vi "Pick Up Order.vi"(8 "error in (no error)":errorcluster, 10 "Beverage":refnum<class "Beverage.lvclass">, 11 "Stub Pick Up Order In":refnum<class "Stub Pick Up Order.lvclass">) -> (0 "error out":errorcluster, 3 "Stub Pick Up Order Out":refnum<class "Stub Pick Up Order.lvclass">)   [LabVIEW 2020, in "Stub Pick Up Order.lvclass"]
uses:
  Stub Pick Up Order.lvclass
  Support/Beverages/Beverage/Beverage.lvclass
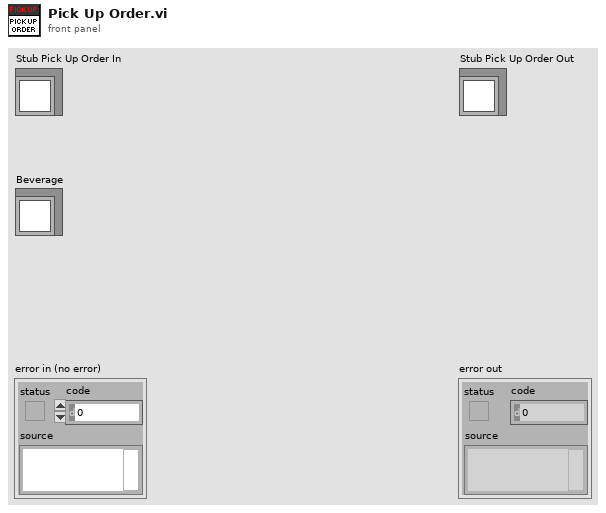
[diagram p1: front panel]
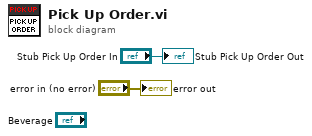
[diagram p0: block diagram]
diagram:
  "error out" <- "error in (no error)"
  "Stub Pick Up Order Out" <- "Stub Pick Up Order In"
